vi "CHROMA Set Current Range.vi"(8 "Error In":errorcluster, 11 "CHROMA VISA In":refnum<visa-resource-name>) -> (0 "Error Out":errorcluster, 3 "CHROMA VISA Out":refnum<visa-resource-name>)   [LabVIEW 2020]
uses:
  Type Definition/CHROMA Build CMD Type.ctl
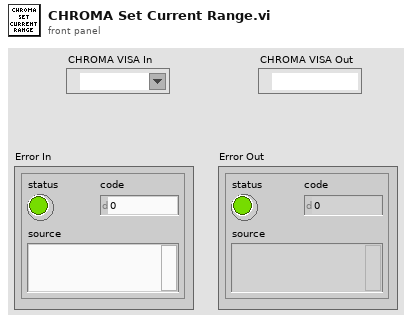
[diagram p1: front panel]
types:
  T1 = typedef "CHROMA Build CMD Type.ctl" = enum16{"Value DBL", "Value I32", "String"}
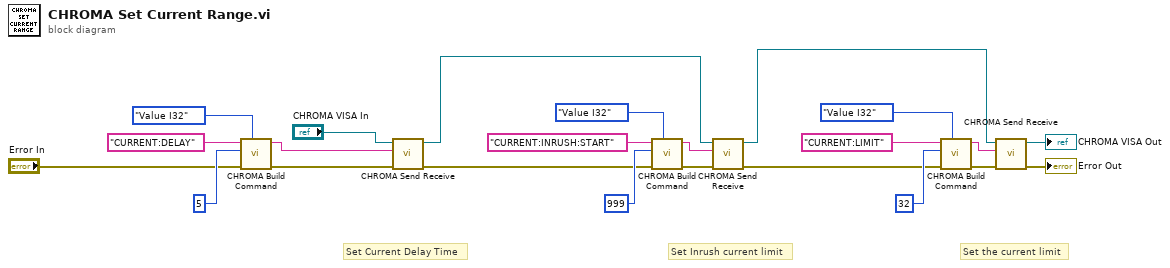
[diagram p0: block diagram]
diagram:
  # "Set the current limit"
  # "Set Inrush current limit"
  # "Set Current Delay Time"
  n1 = call "CHROMA Build Command.vi"("Build Type"=CHROMA_Build_CMD_Type."Value I32", "Error In"="Error In", "Value"=5, "Partial Command"="CURRENT:DELAY" ("string to write")) -> ("Error Out"=w21:errorcluster, "Chroma Command"=w20:string)  [unwired: 6 in]
  n2 = call "CHROMA Send Receive.vi"("error in (no error)"=w21, "Send Command"=w20, "CHROMA VISA In"="CHROMA VISA In") -> ("error out"=w15:errorcluster, "CHROMA VISA Out"=w6:refnum<visa-resource-name>)  [unwired: 6 in, 1 out]
  n3 = call "CHROMA Build Command.vi"("Build Type"=CHROMA_Build_CMD_Type."Value I32", "Error In"=w15, "Value"=999, "Partial Command"="CURRENT:INRUSH:START" ("string to write")) -> ("Error Out"=w17:errorcluster, "Chroma Command"=w18:string)  [unwired: 6 in]
  n4 = call "CHROMA Send Receive.vi"("error in (no error)"=w17, "Send Command"=w18, "CHROMA VISA In"=w6) -> ("error out"=w10:errorcluster, "CHROMA VISA Out"=w7:refnum<visa-resource-name>)  [unwired: 6 in, 1 out]
  n5 = call "CHROMA Build Command.vi"("Build Type"=CHROMA_Build_CMD_Type."Value I32", "Error In"=w10, "Value"=32, "Partial Command"="CURRENT:LIMIT" ("string to write")) -> ("Error Out"=w12:errorcluster, "Chroma Command"=w11:string)  [unwired: 6 in]
  n6 = call "CHROMA Send Receive.vi"("error in (no error)"=w12, "Send Command"=w11, "CHROMA VISA In"=w7) -> ("error out"=→"Error Out":errorcluster, "CHROMA VISA Out"=→"CHROMA VISA Out":refnum<visa-resource-name>)  [unwired: 6 in, 1 out]
